vi "Optics_LoadConfig.vi"(8 "error in (no error)":errorcluster, 11 "Optics config IN":T1={"VISA"="COM3", "Motor numbers"=[7, 8]}) -> (0 "error out":errorcluster, 3 "Optics config OUT":T1={"VISA"="COM3", "Motor numbers"=[]})   [LabVIEW 2021]
doc: "Attempts to load previous user specified settings from an XML file.\n\nThis VI will not generate an error. If a suitable XML file can't be loaded and parsed then it will simply return the default settings."
uses:
  Controls/OpticsConfig.ctl
  <vilib>/Utility/xml.llb/Read From XML File(string).vi
  <vilib>/Utility/xml.llb/Write to XML File(string).vi
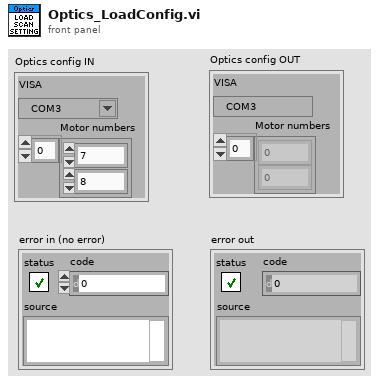
[diagram p1: front panel]
types:
  T1 = typedef "OpticsConfig.ctl" = cluster{"VISA":refnum<visa-resource-name>, "Motor numbers":i32[]}
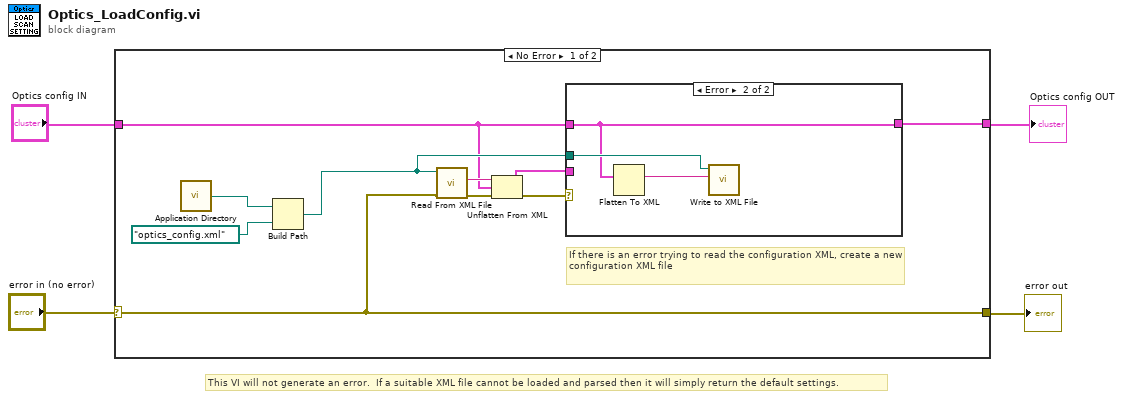
[diagram p0: block diagram]
diagram:
  # "This VI will not generate an error.  If a suitable XML file cannot be loaded and parsed then it will simply return the default settings."
  n1 = case shown="No Error" "error in (no error)" {
    selector: "error in (no error)" -> [w8 w20]
    tunnel: [w8 w20] -> w3
    tunnel: "Optics config IN" -> [w6 w19]
    tunnel: [w7 w19] -> w1
    frame No Error {
      # "If there is an error trying to read the configuration XML, create a new configuration XML file"
      n2 = call <vilib>:"Application Directory.vi"() -> ("Application Directory"=w11:path)
      n3 = Build Path(base path=w11, name or relative path=path "optics_config.xml" ("string")) -> (appended path=w9:path)
      n4 = call-poly <vilib>:"Read From XML File.vi"("error in (no error)"=w8, "XML File Path"=w9) -> ("error out"=w13:errorcluster, "XML Elements"=w14:string)  [unwired: 7 in, 1 out]
      n5 = Unflatten From XML(xml string=w14, type=w6, error in (no error)=w13) -> (value=w5:T1, error out=w12:errorcluster)
      n6 = case shown="Error" w12 {
        tunnel: w5 -> [w15 _]
        tunnel: w9 -> [_ w17]
        tunnel: [w15 w16] -> w7
        tunnel: w6 -> [_ w16]
        frame No Error {
        }
        frame Error {
          n7 = Flatten To XML(6:w16) -> (2:w18:string)
          n8 = call-poly <vilib>:"Write to XML File.vi"("XML Input"=w18, "XML File Path"=w17) -> ()  [unwired: 7 in, 3 out]
        }
      }
    }
    frame Error {
    }
  }
  "error out" <- w3
  "Optics config OUT" <- w1
